vi "Diagnostic Data Lookup Table.vi"(5 "Internal Command Engine References":T2, 6 "command":T3=enum."Get All", 7 "Name":string, 8 "error in (no error)":errorcluster {"code" min=0 max=0}, 9 "Signals":dbl[](array[numeric]), 10 "Signal In":dbl, 11 "Diag Data Ref":T1) -> (0 "error out":errorcluster {"code" min=0 max=0}, 1 "Signals Out":dbl[](array[numeric]), 2 "Signal Out":dbl, 3 "Diag Data Ref out":T1)   [LabVIEW 2015, in "J1939 Addon Engine.lvlib"]
uses:
  J1939 Addon Engine.lvlib
  Types/Diagnostic Data Lookup Table Action.ctl
  Shared/Types/SysDef Command Settings.ctl
  Types/Diagnostic Data Lookup Table Reference.ctl
  Types/Diagnostic Data Lookup Table State Variables.ctl
  Shared/J1939 Addon Shared.lvlib
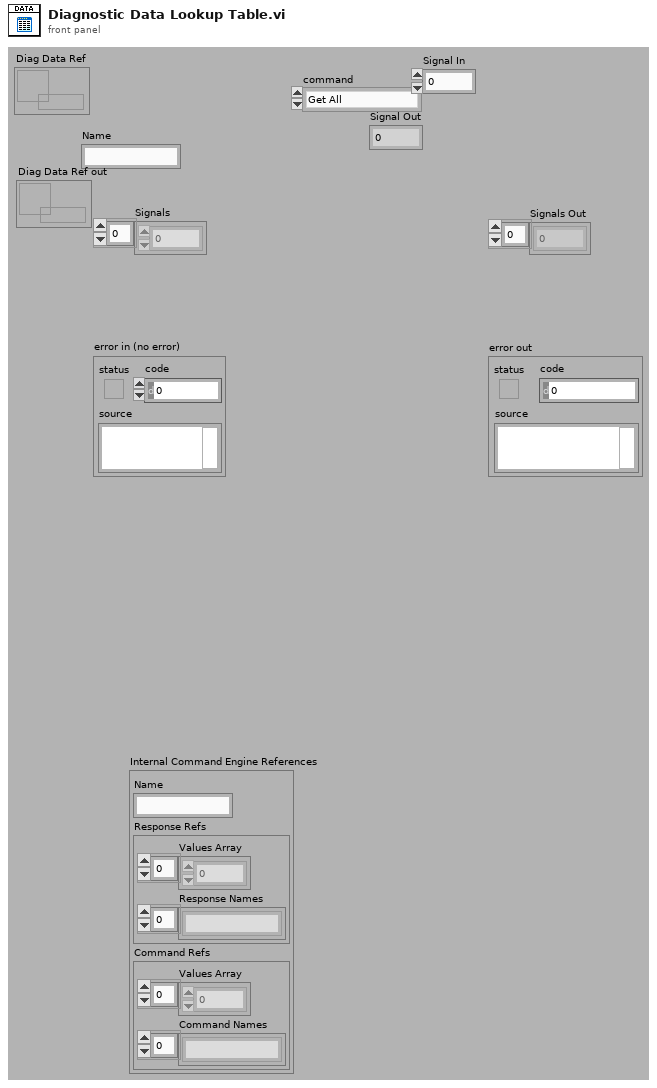
[diagram p1: front panel]
types:
  T1 = typedef "J1939 Addon Engine.lvlib/Diagnostic Data Lookup Table Reference.ctl" = refnum<data-value>
  T2 = typedef "J1939 Addon Shared.lvlib/SysDef Command Settings.ctl" = cluster{"Name":string, "Response Refs":cluster{"Values Array":dbl[], "Response Names":string[]}, "Command Refs":cluster{"Values Array":dbl[], "Command Names":string[]}}
  T3 = typedef "J1939 Addon Engine.lvlib/Diagnostic Data Lookup Table Action.ctl" = enum16{"Initialize", "Get All", "Set All", "Set Value", "Get Value"}
  T4 = typedef "J1939 Addon Engine.lvlib/Diagnostic Data Lookup Table State Variables.ctl" = cluster{"LUT":variant, "Response Names":string[], "Command Names":string[]}
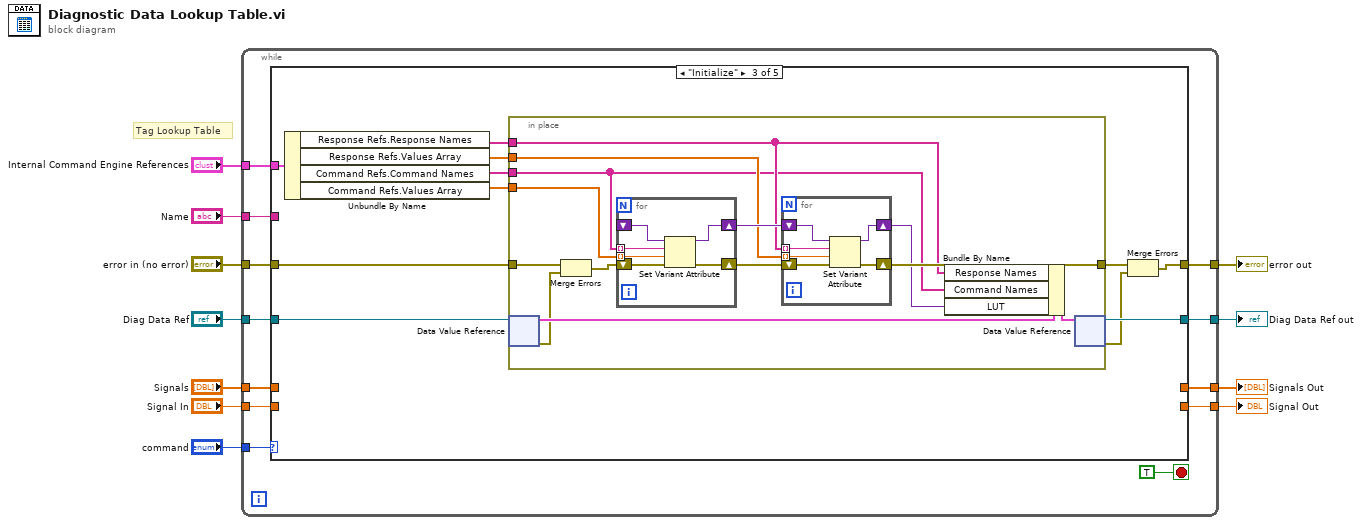
[diagram p0: block diagram]
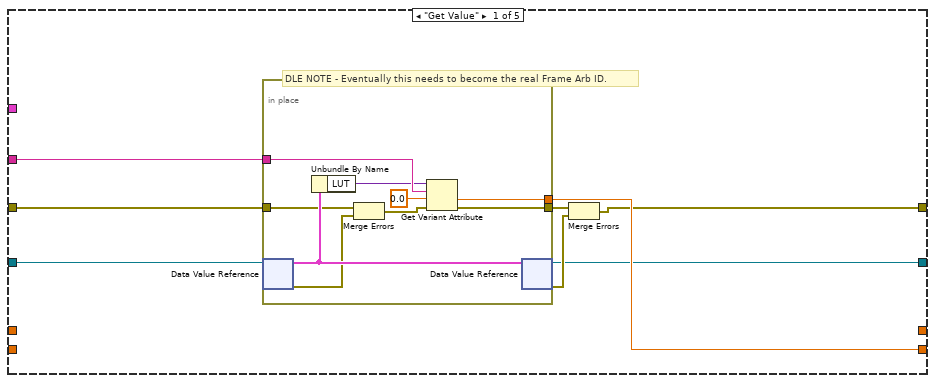
[diagram p2: hidden frame]
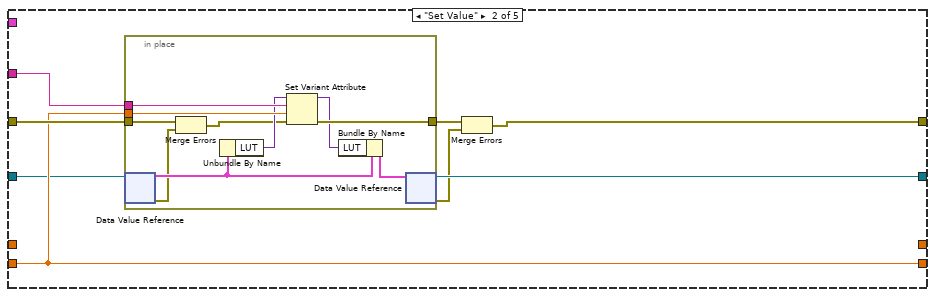
[diagram p3: hidden frame]
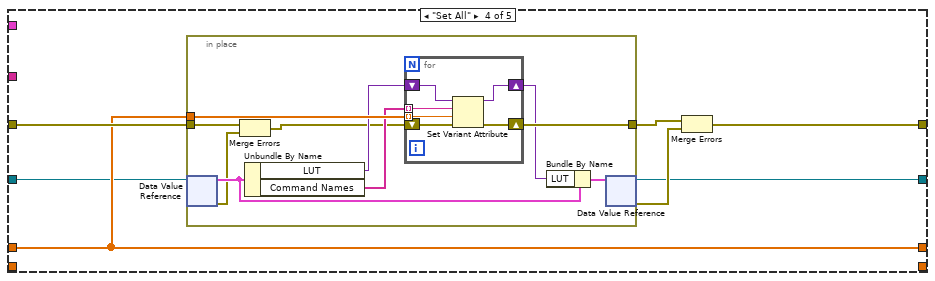
[diagram p4: hidden frame]
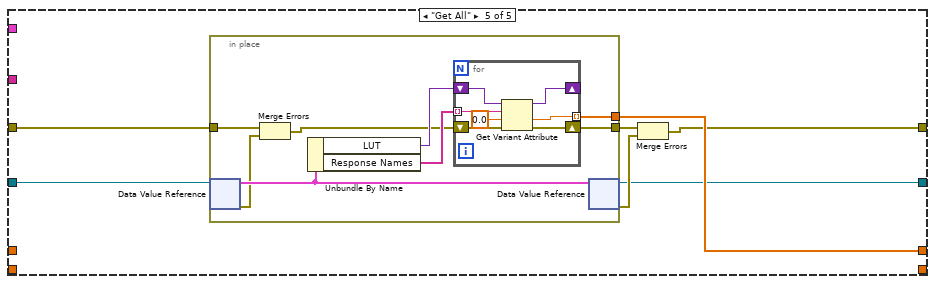
[diagram p5: hidden frame]
diagram:
  # "Tag Lookup Table"
  n1 = while {
    tunnel: "command" -> [w22]
    tunnel: "error in (no error)" -> [w21]
    tunnel: [w20] -> w9
    tunnel: "Name" -> [w19]
    tunnel: "Internal Command Engine References" -> [w18]
    tunnel: [w17] -> w5
    tunnel: "Signals" -> [w16]
    tunnel: [w15] -> w4
    tunnel: "Signal In" -> [w14]
    tunnel: "Diag Data Ref" -> [w13]
    tunnel: [w12] -> w1
    stop <- TRUE stop-if-true
    n2 = case shown="\"Initialize\"" w22 {
      tunnel: w21 -> [w31 w48 w69 w101 w124]
      tunnel: [w26 w42 w60 w97 w120] -> w20
      tunnel: w19 -> [w30 w47 _ _ _]
      tunnel: w18 -> [_ _ w68 _ _]
      tunnel: [_ _ _ w100 w123] -> w17
      tunnel: w16 -> [_ _ _ w100 _]
      tunnel: [w29 w46 _ _ _] -> w15
      tunnel: w14 -> [_ w46 _ _ _]
      tunnel: w13 -> [w28 w45 w63 w99 w122]
      tunnel: [w24 w44 w62 w95 w118] -> w12
      frame "Get Value" {
        # "DLE NOTE - Eventually this needs to become the real Frame Arb ID."
        n3 = in-place {
          in-place-border: w31 -> [w33]
          in-place-border: [w40] -> w25
          in-place-border: w30 -> [w38]
          in-place-border: [w37] -> w29
          n4 = in-place-dvr #1(w28) -> (w35:T4, w34:errorcluster)
          n5 = Unbundle By Name(w35) -> ("LUT"=w36:variant)
          n6 = Merge Errors(w33, w34) -> (w32:errorcluster)
          n7 = Get Variant Attribute(Variant=w36, name=w38, default value (empty Variant)=0.0, error in=w32) -> (value=w37:dbl, error out=w40:errorcluster)  [unwired: 2 out]
          n8 = in-place-dvr #1(w35) -> (w24:T1, w27:errorcluster)
        }
        n9 = Merge Errors(w25, w27) -> (w26:errorcluster)
      }
      frame "Set Value" {
        n10 = in-place {
          in-place-border: w48 -> [w58]
          in-place-border: [w57] -> w41
          in-place-border: w47 -> [w56]
          in-place-border: w46 -> [w55]
          n11 = in-place-dvr #2(w45) -> (w53:T4, w49:errorcluster)
          n12 = Merge Errors(w58, w49) -> (w50:errorcluster)
          n13 = Unbundle By Name(w53) -> ("LUT"=w54:variant)
          n14 = Set Variant Attribute(Variant=w54, name=w56, value=w55, error in=w50) -> (Variant out=w51:variant, error out=w57:errorcluster)  [unwired: 1 out]
          n15 = Bundle By Name(cluster=w53, "LUT"=w51) -> (w52:T4)
          n16 = in-place-dvr #2(w52) -> (w44:T1, w43:errorcluster)
        }
        n17 = Merge Errors(w41, w43) -> (w42:errorcluster)
      }
      frame "Initialize" {
        n18 = Unbundle By Name(w68) -> ("Response Refs.Response Names"=w65:string[], "Response Refs.Values Array"=w66:dbl[], "Command Refs.Command Names"=w64:string[], "Command Refs.Values Array"=w67:dbl[])
        n19 = in-place {
          in-place-border: w69 -> [w71]
          in-place-border: [w80] -> w59
          in-place-border: w67 -> [w79]
          in-place-border: w66 -> [w78]
          in-place-border: w65 -> [w75]
          in-place-border: w64 -> [w74]
          n20 = in-place-dvr #3(w63) -> (w77:T4, w72:errorcluster)
          n21 = Merge Errors(w71, w72) -> (w70:errorcluster)
          n22 = for {
            shift-right: [w93] -> w81
            shift-left: _ -> [w94]
            shift-right: [w91] -> w82
            shift-left: w70 -> [w92]
            tunnel: w74 -> [w90] mode=indexing
            tunnel: w79 -> [w89] mode=indexing
            n23 = Set Variant Attribute(Variant=w94, name=w90, value=w89, error in=w92) -> (Variant out=w93:variant, error out=w91:errorcluster)  [unwired: 1 out]
          }
          n24 = for {
            shift-right: [w87] -> w76
            shift-left: w81 -> [w88]
            shift-right: [w85] -> w80
            shift-left: w82 -> [w86]
            tunnel: w78 -> [w84] mode=indexing
            tunnel: w75 -> [w83] mode=indexing
            n25 = Set Variant Attribute(Variant=w88, name=w83, value=w84, error in=w86) -> (Variant out=w87:variant, error out=w85:errorcluster)  [unwired: 1 out]
          }
          n26 = Bundle By Name(cluster=w77, "Response Names"=w75, "Command Names"=w74, "LUT"=w76) -> (w73:T4)
          n27 = in-place-dvr #3(w73) -> (w62:T1, w61:errorcluster)
        }
        n28 = Merge Errors(w59, w61) -> (w60:errorcluster)
      }
      frame "Set All" {
        n29 = in-place {
          in-place-border: [w111] -> w96
          in-place-border: w101 -> [w103]
          in-place-border: w100 -> [w110]
          n30 = in-place-dvr #4(w99) -> (w107:T4, w104:errorcluster)
          n31 = Merge Errors(w103, w104) -> (w102:errorcluster)
          n32 = Unbundle By Name(w107) -> ("LUT"=w109:variant, "Command Names"=w108:string[])
          n33 = for {
            shift-right: [w116] -> w106
            shift-left: w109 -> [w117]
            shift-right: [w114] -> w111
            shift-left: w102 -> [w115]
            tunnel: w110 -> [w113] mode=indexing
            tunnel: w108 -> [w112] mode=indexing
            n34 = Set Variant Attribute(Variant=w117, name=w112, value=w113, error in=w115) -> (Variant out=w116:variant, error out=w114:errorcluster)  [unwired: 1 out]
          }
          n35 = Bundle By Name(cluster=w107, "LUT"=w106) -> (w105:T4)
          n36 = in-place-dvr #4(w105) -> (w95:T1, w98:errorcluster)
        }
        n37 = Merge Errors(w96, w98) -> (w97:errorcluster)
      }
      frame "Get All" {
        n38 = in-place {
          in-place-border: w124 -> [w126]
          in-place-border: [w132] -> w119
          in-place-border: [w131] -> w123
          n39 = in-place-dvr #5(w122) -> (w128:T4, w127:errorcluster)
          n40 = Merge Errors(w126, w127) -> (w125:errorcluster)
          n41 = Unbundle By Name(w128) -> ("LUT"=w130:variant, "Response Names"=w129:string[])
          n42 = for {
            shift-right: [w138] -> _
            shift-left: w130 -> [w139]
            shift-right: [w136] -> w132
            shift-left: w125 -> [w137]
            tunnel: w129 -> [w135] mode=indexing
            tunnel: [w133] -> w131 mode=indexing
            n43 = Get Variant Attribute(Variant=w139, name=w135, default value (empty Variant)=0.0, error in=w137) -> (duplicate Variant=w138:variant, value=w133:dbl, error out=w136:errorcluster)  [unwired: 1 out]
          }
          n44 = in-place-dvr #5(w128) -> (w118:T1, w121:errorcluster)
        }
        n45 = Merge Errors(w119, w121) -> (w120:errorcluster)
      }
    }
  }
  "error out" <- w9
  "Signals Out" <- w5
  "Signal Out" <- w4
  "Diag Data Ref out" <- w1
